vi "ReadData.vi"(10 "Port name":string, 11 "Reference ID":u64) -> (0 "Error code":i32, 2 "Port data":u8, 3 "Reference ID out":u64)   [LabVIEW 2023]
doc: "Reads data from a specific channel mentioned."
uses:
  <vilib>/Utility/error.llb/Error Cluster From Error Code.vi
  <vilib>/rvi/errors/niLvFpgaAdjustHostInterfaceError.vi
  <vilib>/rvi/interface/nirviReadWriteControl/nirviReadWriteControl.xnode
  NiFpgaLv.dll
  <vilib>/rvi/interface/Simulation/niFpgaSimulationCallBeginRW.vi
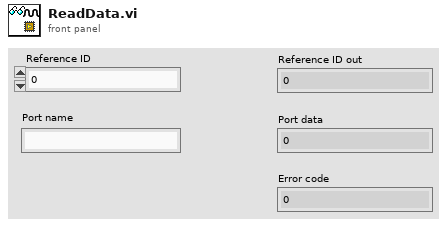
[diagram p1: front panel]
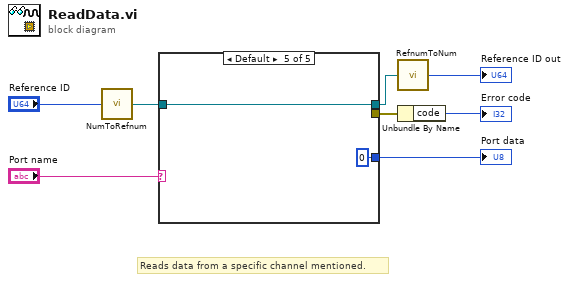
[diagram p0: block diagram]
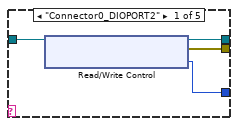
[diagram p2: hidden frame]
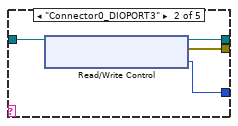
[diagram p3: hidden frame]
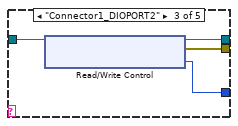
[diagram p4: hidden frame]
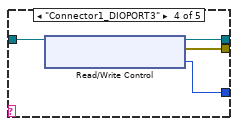
[diagram p5: hidden frame]
diagram:
  # "Reads data from a specific channel mentioned."
  n1 = call "NumToRefnum.vi"("Reference ID"="Reference ID") -> ("Refnum Out"=w8:refnum<k20>)
  n2 = case shown="Default" "Port name" {
    tunnel: w8 -> [w12 w16 w20 w24 w26]
    tunnel: [w11 w15 w19 w23 w26] -> w7
    tunnel: [w10 w14 w18 w22 _] -> w4
    tunnel: [w9 w13 w17 w21 u8 0 ("Connector1/DIOPORT0")] -> w3
    frame "Connector0_DIOPORT2" {
      n3 = xnode ("Read/Write Control")("FPGA VI Reference In"=w12) -> ("FPGA VI Reference Out"=w11:refnum<k20>, "error out"=w10:errorcluster, "Connector 0/DIOPORT2"=w9:u8)  [unwired: 1 in]
    }
    frame "Connector0_DIOPORT3" {
      n4 = xnode ("Read/Write Control")("FPGA VI Reference In"=w16) -> ("FPGA VI Reference Out"=w15:refnum<k20>, "error out"=w14:errorcluster, "Connector 0/DIOPORT3"=w13:u8)  [unwired: 1 in]
    }
    frame "Connector1_DIOPORT2" {
      n5 = xnode ("Read/Write Control")("FPGA VI Reference In"=w20) -> ("FPGA VI Reference Out"=w19:refnum<k20>, "error out"=w18:errorcluster, "Connector1/DIOPORT2"=w17:u8)  [unwired: 1 in]
    }
    frame "Connector1_DIOPORT3" {
      n6 = xnode ("Read/Write Control")("FPGA VI Reference In"=w24) -> ("FPGA VI Reference Out"=w23:refnum<k20>, "error out"=w22:errorcluster, "Connector1/DIOPORT3"=w21:u8)  [unwired: 1 in]
    }
    frame Default {
    }
  }
  "Port data" <- w3
  n7 = call "RefnumToNum.vi"("Refnum in"=w7) -> ("Reference ID"=→"Reference ID out":u64)
  n8 = Unbundle By Name(w4) -> ("code"=→"Error code":i32)
